vi "AL_Rotate_mouse_coords.vi"(1 "Mouse angle of rotation, deg":dbl, 2 "Offset":T1, 3 "Coordinates to rotate":T1) -> (0 "Rotated coordinates":cluster{"X":dbl, "Y":dbl})   [LabVIEW 2016]
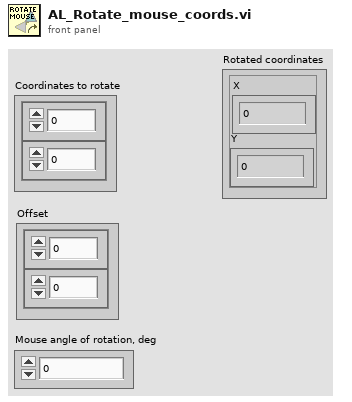
[diagram p1: front panel]
types:
  T1 = cluster{"Numeric Control":dbl, "Numeric Control":dbl}
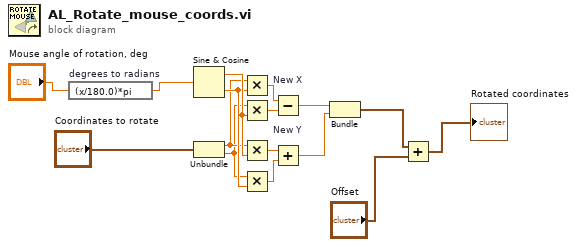
[diagram p0: block diagram]
diagram:
  n1 = expression code="(x/180.0)*pi" "degrees to radians"("Mouse angle of rotation, deg") -> (w4:dbl)
  n2 = Sine & Cosine(0:w4) -> (1:w13:dbl, 2:w12:dbl)
  n3 = Unbundle("Coordinates to rotate") -> ("Numeric Control"=w9:dbl, "Numeric Control"=w8:dbl)
  n4 = Multiply(x=w9, y=w12) -> (x*y=w15:dbl)
  n5 = Multiply(x=w8, y=w13) -> (x*y=w14:dbl)
  n6 = Multiply(x=w9, y=w13) -> (x*y=w11:dbl)
  n7 = Multiply(x=w8, y=w12) -> (x*y=w10:dbl)
  n8 = Subtract "New X"(x=w15, y=w14) -> (x-y=w7:dbl)
  n9 = Add "New Y"(x=w11, y=w10) -> (x+y=w6:dbl)
  n10 = Bundle(w7, w6) -> (w2:cluster{dbl, dbl})  [unwired: 1 in]
  n11 = Add(x=w2, y="Offset") -> (x+y=→"Rotated coordinates":cluster{dbl, dbl})
